vi "draw.vi"(0 "reference":refnum<class "InitialStateNode.lvclass">, 1 "graphics":refnum<class "Graphics.lvclass">, 5 "error in (no error)":errorcluster) -> (14 "reference out":refnum<class "InitialStateNode.lvclass">, 19 "error out":errorcluster)   [LabVIEW 2020, in "InitialStateNode.lvclass"]
doc: "public void draw(Graphics2D g2, Point2D p, Point2D q)"
uses:
  <resource>/Framework/Providers/Open_GDS/UML/InitialStateNode_class/InitialStateNode.lvclass
  C:/Program Files (x86)/National Instruments/LabVIEW 2020/resource/Framework/Providers/Open_GDS/UML/RectangularNode_class/RectangularNode.lvclass
  <resource>/Framework/Providers/Open_GDS/UML/Graphics_class/Graphics.lvclass
  <resource>/Framework/Providers/Open_GDS/UML/MultiLineString_class/MultiLineString.lvclass
  <resource>/Framework/Providers/Open_GDS/UML/RectangularNode_class/RectangularNode.lvclass
panel:
  in  "Case Constant\n(See Context Help)":bool
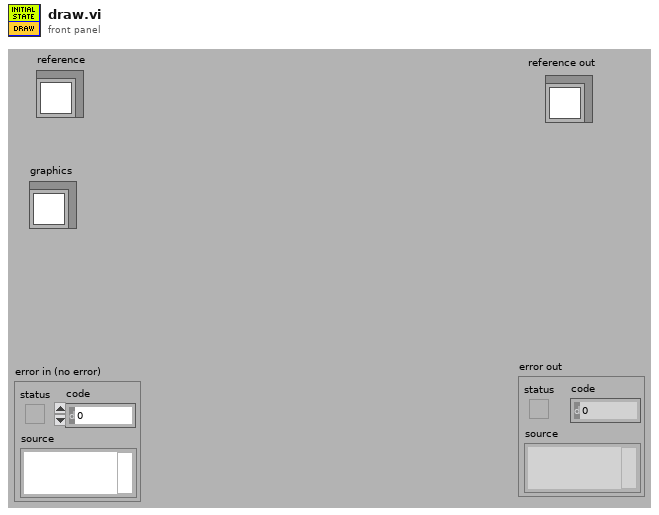
[diagram p1: front panel]
types:
  T1 = typedef "InitialStateNode.lvclass/ObjectAttributes.ctl" = cluster{"name":refnum<class "MultiLineString.lvclass">, "DEFAULT_WIDTH":i32, "DEFAULT_HEIGHT":i32}
  T2 = typedef "RectangularNode.lvclass/ObjectAttributes.ctl" = cluster{"bounds":T3}
  T3 = typedef "Rectangle Rectangle2D.ctl" = cluster{"x":dbl, "y":dbl, "width":dbl, "height":dbl}
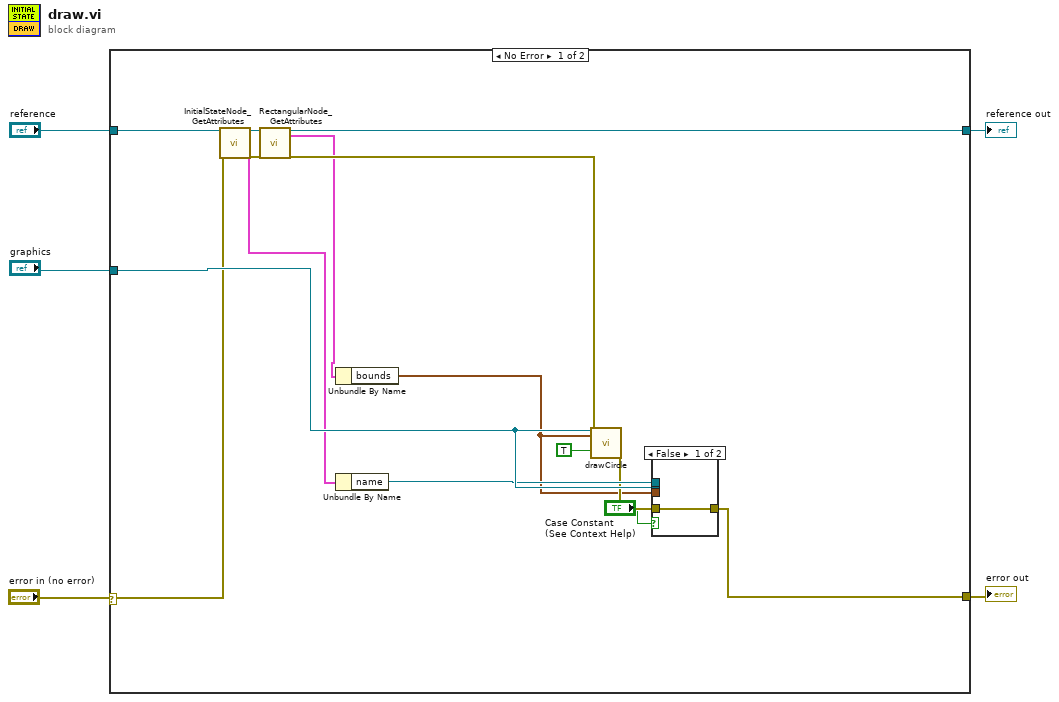
[diagram p0: block diagram]
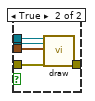
[diagram p2: hidden frame]
diagram:
  n1 = case shown="No Error" "error in (no error)" {
    selector: "error in (no error)" -> [w14 w27]
    tunnel: "reference" -> [w20 w28]
    tunnel: [w19 w27] -> w4
    tunnel: [w7 w28] -> w3
    tunnel: "graphics" -> [w18 _]
    frame No Error {
      n2 = call <resource>:"InitialStateNode_GetAttributes.vi"("reference in"=w20, "error in (no error)"=w14) -> ("reference out"=w10:refnum<class "InitialStateNode.lvclass">, "Data"=w11:T1, "error out"=w9:errorcluster)  [unwired: 1 in, 14 out]
      n3 = call <resource>:"RectangularNode_GetAttributes.vi"("reference in"=w10, "error in (no error)"=w9) -> ("reference out"=w7:refnum<class "InitialStateNode.lvclass">, "Data"=w6:T2, "error out"=w8:errorcluster)  [unwired: 14 in, 1 out]
      n4 = Unbundle By Name(w6) -> ("bounds"=w15:T3)
      n5 = Unbundle By Name(w11) -> ("name"=w17:refnum<class "MultiLineString.lvclass">)
      n6 = call-dynamic "drawCircle.vi"("reference"=w18, "rectangle"=w15, "fill?(F)"=TRUE, "error in (no error)"=w8) -> ("error out"=w16:errorcluster)  [unwired: 14 in, 1 out]
      n7 = case shown="False" "Case Constant\n(See Context Help)" {
        tunnel: [w21 w26] -> w19
        tunnel: w18 -> [_ w25]
        tunnel: w17 -> [_ w24]
        tunnel: w16 -> [w21 w23]
        tunnel: w15 -> [_ w22]
        frame False {
        }
        frame True {
          n8 = call-dynamic "draw.vi"("reference"=w24, "graphics"=w25, "bounds"=w22, "error in (no error)"=w23) -> ("error out"=w26:errorcluster)  [unwired: 14 in, 1 out]
        }
      }
    }
    frame Error {
    }
  }
  "reference out" <- w3
  "error out" <- w4
